vi "图像采集template.vi"() -> ()   [LabVIEW 2018]
uses:
  <vilib>/userdefined/High Color/IMAQdx.ctl
panel:
  in  "Session In":T1
  out "Image":T2(plugin-control)
  in  "安全退出":bool
  in  "采集图像":bool
  in  "打开摄像头":bool
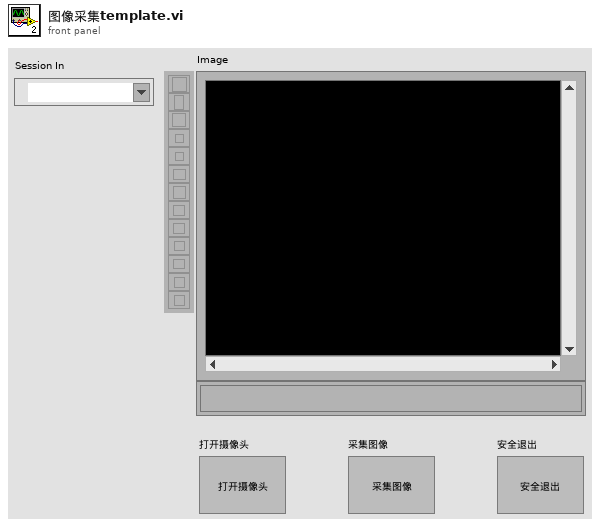
[diagram p1: front panel]
types:
  T1 = typedef "IMAQdx.ctl" = refnum<k21>
  T2 = typedef "IMAQ Image.ctl" = refnum<image>
  T3 = typedef "控件 1.ctl" = string
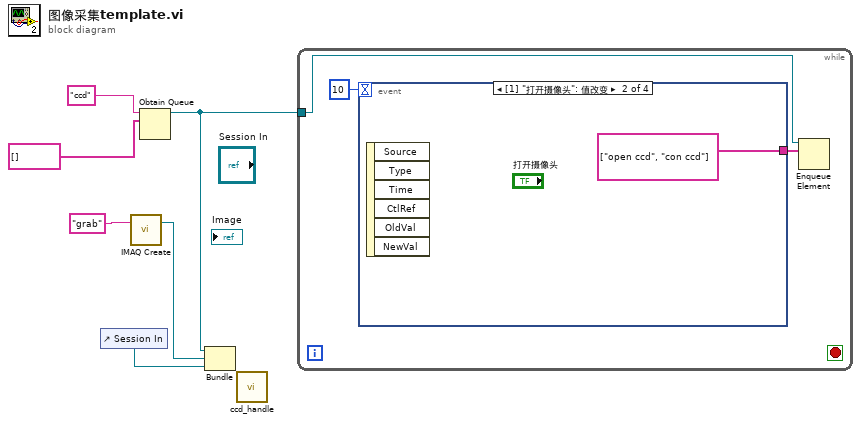
[diagram p0: block diagram]
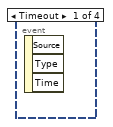
[diagram p2: hidden frame]
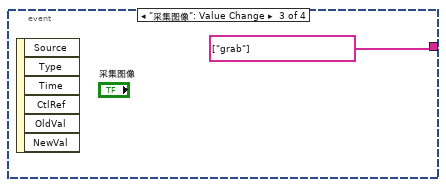
[diagram p3: hidden frame]
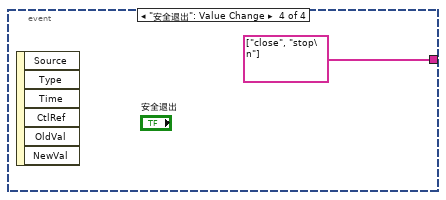
[diagram p4: hidden frame]
diagram:
  n1 = control-ref of="Session In"() -> (w1:refnum<vi>)
  n2 = call "IMAQ Create"("Image Name"="grab") -> ("New Image"=w2:T2)  [unwired: 4 in, 1 out]
  n3 = Obtain Queue(name (unnamed)="ccd", element data type=string[] [] ("添加的数组")) -> (queue out=w3:refnum<queue>)  [unwired: 3 in, 2 out]
  n4 = Bundle("queue out"=w3, "New Image"=w2, "Session In"=w1) -> ()  [unwired: 1 in, 1 out]
  n5 = call "ccd_handle.vi"() -> ()  [unwired: 12 in]
  n6 = while {
    tunnel: w3 -> [w8]
    stop <- _ stop-if-true
    n7 = event shown="[1] \"打开摄像头\": 值改变" {
      selector: _ -> [_ _ _ _]
      dyn-events: _ -> [_ _ _ _]
      timeout: 10 -> [_ _ _ _]
      tunnel: [_ T3[] ["open ccd", "con ccd"] ("元素") T3[] ["grab"] ("元素") T3[] ["close", "stop\n"] ("元素")] -> w7
      event Timeout {
        n8 = event-data() -> ()  [unwired: 1 in, 3 out]
      }
      event "打开摄像头": Value Change {
        n9 = event-data() -> ()  [unwired: 1 in, 6 out]
      }
      event "采集图像": Value Change {
        n10 = event-data() -> ()  [unwired: 1 in, 6 out]
      }
      event "安全退出": Value Change {
        n11 = event-data() -> ()  [unwired: 1 in, 6 out]
      }
    }
    n12 = Enqueue Element(queue=w8, element=w7) -> ()  [unwired: 2 in, 3 out]
  }
